vi "PolConfig.vi"() -> ()   [LabVIEW 2009]
doc: "Configures the Polhemus Fastrak for use. Can change units, output format, output contents.\nAllows saving to the EEPROM which saves the state of the configuration when the power is cycled on the Polhemus."
uses:
  BaudRateSelector.ctl
  <vilib>/Instr/_visa.llb/VISA Configure Serial Port (Instr).vi
panel:
  in  "stop":bool
  in  "Configure Button":bool
  out "Output":string
  in  "Input":string="P"
  in  "Test Configuration?":bool
  in  "Only Send Custom\n(Save Feature still in effect)":bool
  in  "Special Commands":string
  in  "Station Controls":cluster{"Output Listing":u16[]}[](array[cluster])=[{"Output Listing"=[2, 4]}, {"Output Listing"=[2, 4, 1]}] {"Output Listing" items=["Cartesian Coordinates"=2, "Euler Orientation"=4, "ASCII Space"=0, "CR, LF"=1]}
  in  "Save to EEPROM?":bool
  in  "Output Format":enum16{"ASCII", "Binary"}(ring)=enum."Binary"
  in  "Units":enum16{"Inches", "Centimeters"}(ring)=enum."Centimeters"
  in  "Parity":enum16{"None", "Odd", "Even", "Mark", "Space"}(ring)
  in  "Data Bits":u16=8 min=7 max=8 step=1
  in  "Baud Rate":T1=115200 items=["1200"=1200, "2400"=2400, "4800"=4800, "9600"=9600, "19200"=19200, "38400"=38400, "57600"=57600, "115200"=115200]
  in  "VISA resource name":refnum<visa-resource-name>="COM3"
  # "Polhemus 3SPACE FASTRAK Configuration Tool\n~~~~~~~~~"
  # "Basic Serial Information"
  # "Polhemus Settings Config"
  # "Custom Commands to Send"
  # "This tool sends commands to the Polhemus Fastrak to configure it for desired use.\nIn addition to basic status configuration, the output of the receiver functions can be changed here. The 4 most basic commands are listed, however other commands can be issued by typing in the number specified by the manual on pg. 98 to the right of the menu.\nTo remove a command, right-click and select  \"Delete Element\"."
  # "If Data Bits = 8, Parity must be \"None\""
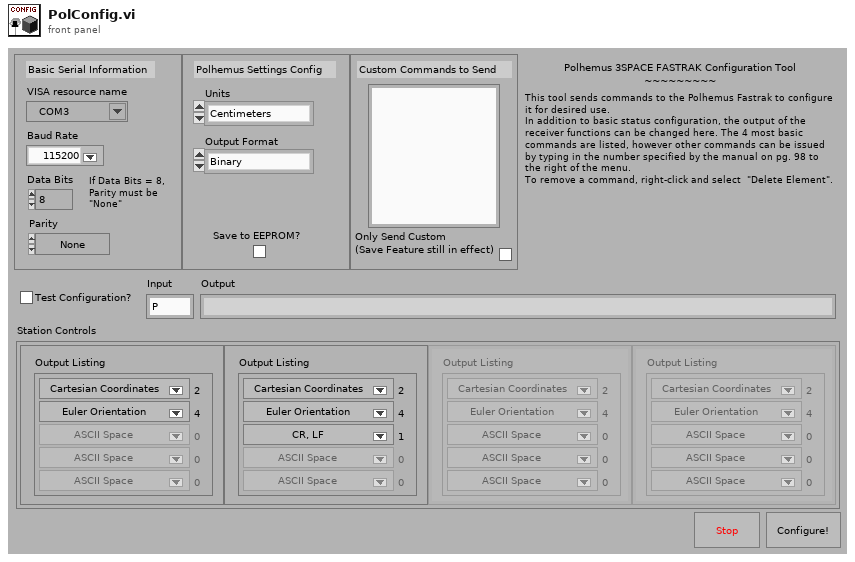
[diagram p1: front panel]
types:
  T1 = typedef "BaudRateSelector.ctl" = u32
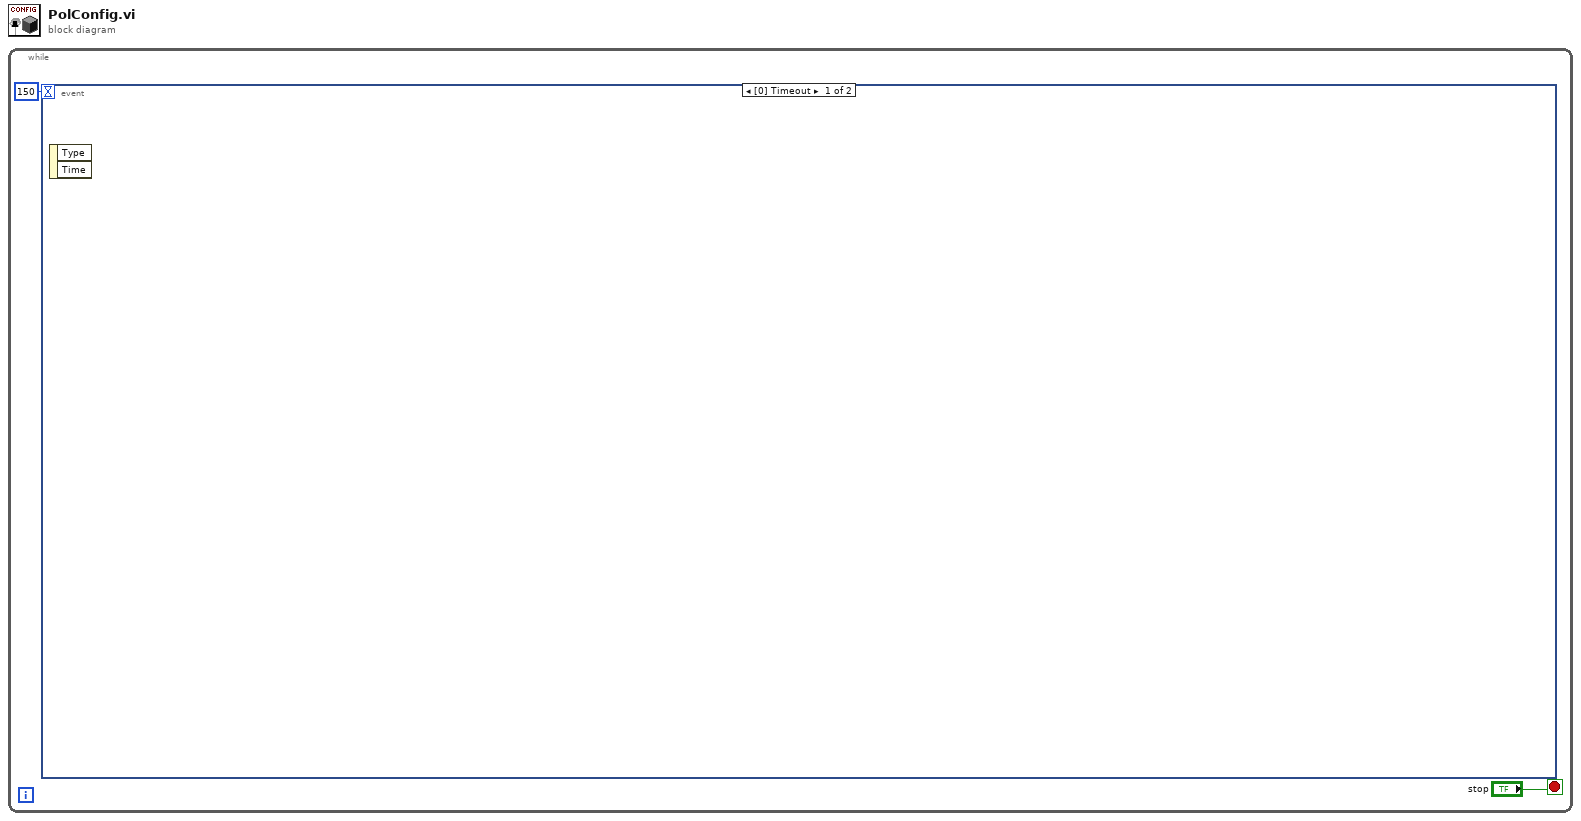
[diagram p0: block diagram]
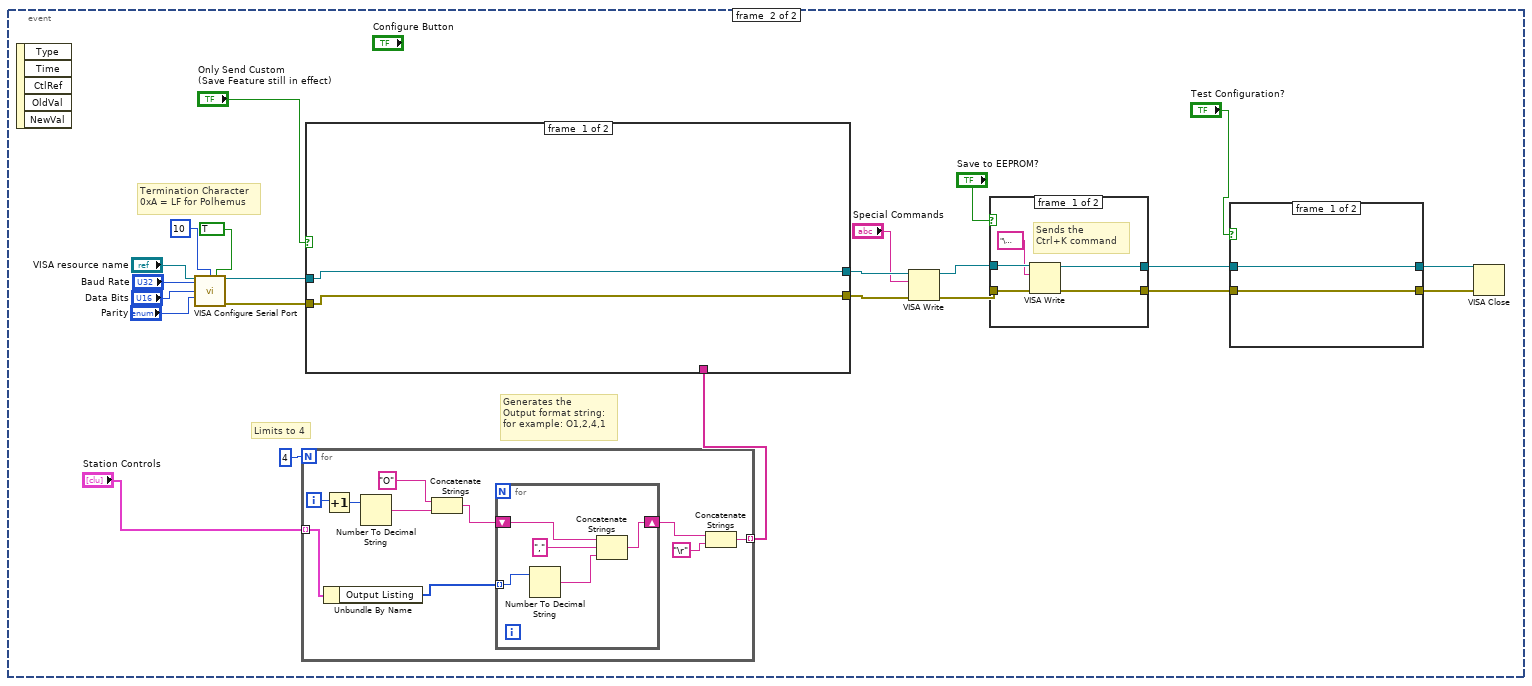
[diagram p2: hidden frame]
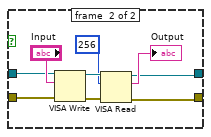
[diagram p3: hidden frame]
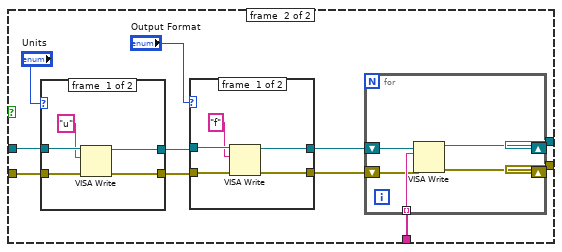
[diagram p4: hidden frame]
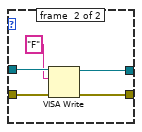
[diagram p5: hidden frame]
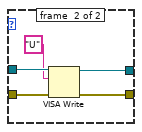
[diagram p6: hidden frame]
diagram:
  n1 = while {
    stop <- "stop" stop-if-true
    n2 = event shown="[0] Timeout" {
      selector: _ -> [_ _]
      dyn-events: _ -> [_ _]
      timeout: 150 -> [_ _]
      event #0 {
        n3 = event-data() -> ()  [unwired: 1 in, 2 out]
      }
      event #1 {
        # "Limits to 4"
        # "Generates the\nOutput format string:\nfor example: O1,2,4,1"
        # "Termination Character\n0xA = LF for Polhemus"
        n4 = event-data() -> ()  [unwired: 1 in, 5 out]
        n5 = call-poly "VISA Configure Serial Port"("VISA resource name"="VISA resource name", "termination char\n(0xA = '\\n' = LF)"=u8 10 ("termination char\n(0xA = '\\n' = LF)"), "Enable Termination\nChar (T)"=TRUE ("Enable Termination\nChar (T)"), "baud rate (9600)"="Baud Rate", "data bits (8)"="Data Bits", "parity (0:none)"="Parity") -> ("VISA resource name out"=w9:refnum<visa-resource-name>, "error out"=w10:errorcluster)  [unwired: 8 in]
        n6 = for {
          N: 4 -> [_]
          tunnel: "Station Controls" -> [w91] mode=indexing
          tunnel: [w86] -> w11 mode=indexing
          i -> [w85]
          n7 = Increment(x=w85) -> (x+1=w84:i32)
          n8 = Unbundle By Name(w91) -> ("Output Listing"=w83:u16[])
          n9 = Number To Decimal String(number=w84) -> (decimal integer string=w89:string)  [unwired: 1 in]
          n10 = Concatenate Strings("O", w89) -> (w88:string)
          n11 = for {
            tunnel: w83 -> [w96] mode=indexing
            shift-right: [w93] -> w87
            shift-left: w88 -> [w95]
            n12 = Number To Decimal String(number=w96) -> (decimal integer string=w92:string)  [unwired: 1 in]
            n13 = Concatenate Strings(w95, ",", w92) -> (w93:string)
          }
          n14 = Concatenate Strings(w87, "\r") -> (w86:string)
        }
        n15 = case shown="False" "Only Send Custom\n(Save Feature still in effect)" {
          tunnel: w9 -> [w38 w48]
          tunnel: w10 -> [w37 w47]
          tunnel: w11 -> [_ w43]
          tunnel: [w38 w40] -> w14
          tunnel: [w37 w39] -> w16
          frame #0 {
          }
          frame #1 {
            n16 = case shown="\"Centimeters\", Default" "Units" {
              tunnel: w48 -> [w68 w73]
              tunnel: w47 -> [w69 w74]
              tunnel: [w66 w71] -> w45
              tunnel: [w65 w70] -> w44
              frame #0 {
                n17 = VISA Write(VISA resource name=w68, write buffer="u", error in (no error)=w69) -> (VISA resource name out=w66:refnum<visa-resource-name>, error out=w65:errorcluster)  [unwired: 1 out]
              }
              frame #1 {
                n18 = VISA Write(VISA resource name=w73, write buffer="U", error in (no error)=w74) -> (VISA resource name out=w71:refnum<visa-resource-name>, error out=w70:errorcluster)  [unwired: 1 out]
              }
            }
            n19 = case shown="\"Binary\", Default" "Output Format" {
              tunnel: w45 -> [w58 w63]
              tunnel: w44 -> [w59 w64]
              tunnel: [w56 w61] -> w41
              tunnel: [w55 w60] -> w42
              frame #0 {
                n20 = VISA Write(VISA resource name=w58, write buffer="f", error in (no error)=w59) -> (VISA resource name out=w56:refnum<visa-resource-name>, error out=w55:errorcluster)  [unwired: 1 out]
              }
              frame #1 {
                n21 = VISA Write(VISA resource name=w63, write buffer="F", error in (no error)=w64) -> (VISA resource name out=w61:refnum<visa-resource-name>, error out=w60:errorcluster)  [unwired: 1 out]
              }
            }
            n22 = for {
              tunnel: w43 -> [w54] mode=indexing
              shift-right: [w51] -> w40
              shift-left: w41 -> [w52]
              shift-right: [w50] -> w39
              shift-left: w42 -> [w53]
              n23 = VISA Write(VISA resource name=w52, write buffer=w54, error in (no error)=w53) -> (VISA resource name out=w51:refnum<visa-resource-name>, error out=w50:errorcluster)  [unwired: 1 out]
            }
          }
        }
        n24 = VISA Write(VISA resource name=w14, write buffer="Special Commands", error in (no error)=w16) -> (VISA resource name out=w15:refnum<visa-resource-name>, error out=w17:errorcluster)  [unwired: 1 out]
        n25 = case shown="True" "Save to EEPROM?" {
          tunnel: w15 -> [w78 w81]
          tunnel: w17 -> [w79 w80]
          tunnel: [w76 w81] -> w20
          tunnel: [w75 w80] -> w21
          frame #0 {
            # "Sends the\nCtrl+K command"
            n26 = VISA Write(VISA resource name=w78, write buffer="\u000b", error in (no error)=w79) -> (VISA resource name out=w76:refnum<visa-resource-name>, error out=w75:errorcluster)  [unwired: 1 out]
          }
          frame #1 {
          }
        }
        n27 = case shown="True" "Test Configuration?" {
          tunnel: w20 -> [w27 w35]
          tunnel: w21 -> [w26 w34]
          tunnel: [w27 w30] -> w22
          tunnel: [w26 w29] -> w23
          frame #0 {
          }
          frame #1 {
            n28 = VISA Write(VISA resource name=w35, write buffer="Input", error in (no error)=w34) -> (VISA resource name out=w33:refnum<visa-resource-name>, error out=w32:errorcluster)  [unwired: 1 out]
            n29 = VISA Read(VISA resource name=w33, byte count=u32 256, error in (no error)=w32) -> (VISA resource name out=w30:refnum<visa-resource-name>, read buffer=→"Output":string, error out=w29:errorcluster)  [unwired: 1 out]
          }
        }
        n30 = VISA Close(VISA resource name=w22, error in (no error)=w23) -> ()  [unwired: 1 out]
      }
    }
  }
